vi "Process Selection.vi"(8 "error in (no error)":errorcluster, 11 "Test Selector in":refnum<class "Test Selector.lvclass">) -> (0 "error out":errorcluster, 3 "Test Selector out":refnum<class "Test Selector.lvclass">)   [LabVIEW 2019, in "Test Selector.lvlib" / "Test Selector.lvclass"]
uses:
  Test Selector.lvclass
  Test Selector.lvclass/Test Selector.ctl
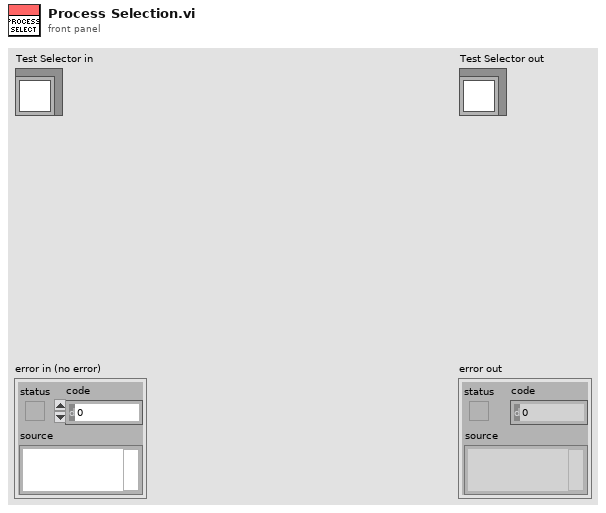
[diagram p1: front panel]
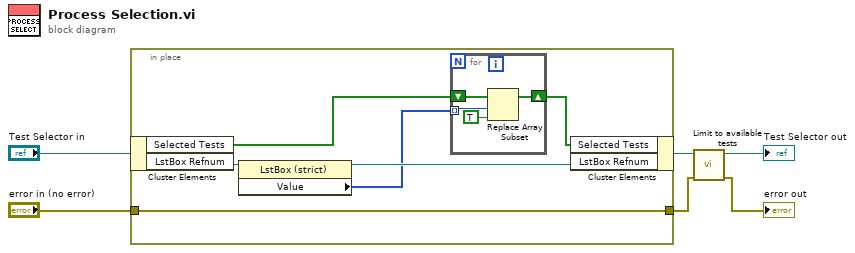
[diagram p0: block diagram]
diagram:
  n1 = in-place {
    in-place-border: "error in (no error)" -> [w10]
    in-place-border: [w10] -> w2
    n2 = in-place-cluster #1("Test Selector in") -> ("Selected Tests"=w9:bool[], "LstBox Refnum"=w12:refnum<vi>)
    n3 = property class="LstBox (strict)"(reference=w12) -> (reference out=w11:refnum<vi>, "Value"=w7:i32[])  [unwired: 1 in, 1 out]
    n4 = for {
      shift-right: [w15] -> w8
      shift-left: w9 -> [w16]
      tunnel: w7 -> [w14] mode=indexing
      n5 = Replace Array Subset(array=w16, new element=TRUE ("new element/subarray"), index=w14) -> (w15:bool[])
    }
    n6 = in-place-cluster #1("Selected Tests"=w8, "LstBox Refnum"=w11) -> (w4:refnum<class "Test Selector.lvclass">)
  }
  n7 = call "Limit to available tests.vi"("error in (no error)"=w2, "Test Selector in"=w4) -> ("error out"=→"error out":errorcluster, "Test Selector out"=→"Test Selector out":refnum<class "Test Selector.lvclass">)  [unwired: 8 in]
